vi "Initialize.vi"(8 "error in (no error)":errorcluster, 11 "Controller Actor.lvlib:Controller.lvclass":refnum<class "Controller.lvclass">) -> (0 "error out":errorcluster, 3 "Controller out":refnum<class "Controller.lvclass">)   [LabVIEW 2016, in "Controller Actor.lvlib" / "Controller.lvclass"]
uses:
  Controller.lvclass
  C:/Program Files (x86)/National Instruments/LabVIEW 2016/vi.lib/ActorFramework/Actor/Actor.lvclass
  <vilib>/ActorFramework/Actor/Actor.lvclass/Actor.ctl
  <vilib>/ActorFramework/Message Enqueuer/Message Enqueuer.lvclass/Message Enqueuer.ctl
  <vilib>/ActorFramework/Message Enqueuer/Init from Existing Queue.vi
  <vilib>/ActorFramework/Message Enqueuer/Enqueue.vi
  Messages/Measurements Scan Msg/Measurements Scan Msg.lvclass
  C:/Program Files (x86)/National Instruments/LabVIEW 2016/vi.lib/ActorFramework/Message/Message.lvclass
  <vilib>/ActorFramework/Message Priority Queue/Priority Enqueue.vi
  <vilib>/ActorFramework/Message Enqueuer/Message Enqueuer.lvclass
  <vilib>/ActorFramework/Actor/Actor.lvclass
  Messages/Scan Hardware Message/Scan Hardware Message.lvclass
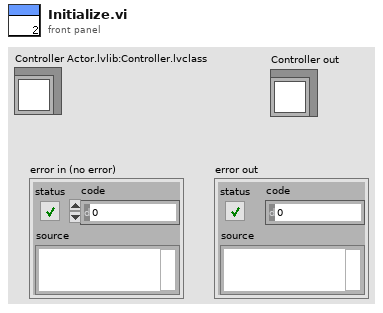
[diagram p1: front panel]
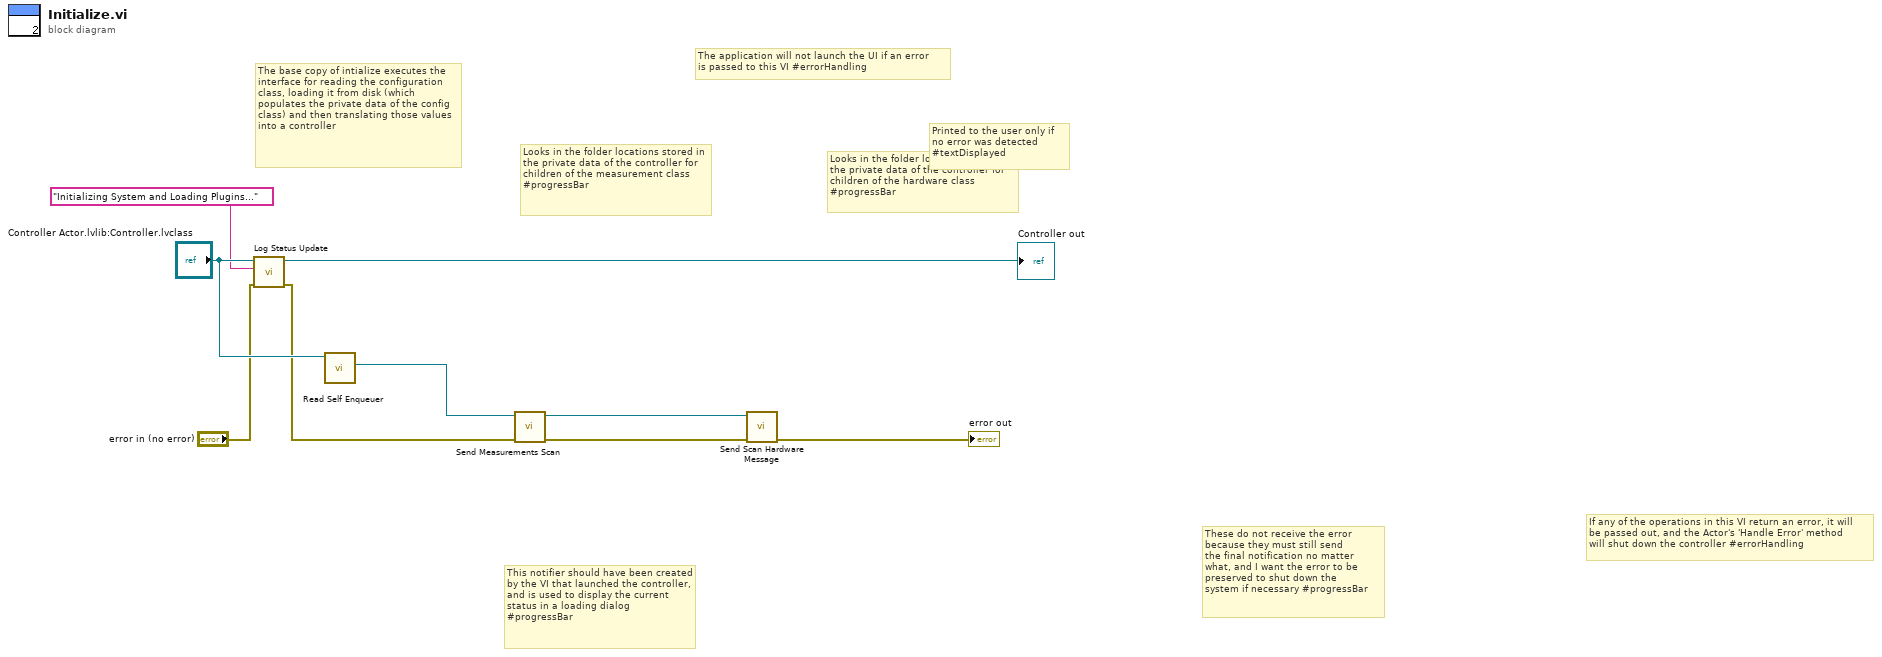
[diagram p0: block diagram]
diagram:
  # "The base copy of intialize executes the interface for reading the configuration class, loading it from disk (which populates the private data of the config class) and then translating those values into a controller"
  # "Printed to the user only if \nno error was detected\n#textDisplayed"
  # "This notifier should have been created by the VI that launched the controller, and is used to display the current status in a loading dialog #progressBar"
  # "Looks in the folder locations stored in the private data of the controller for children of the hardware class \n#progressBar"
  # "Looks in the folder locations stored in the private data of the controller for children of the measurement class #progressBar"
  # "These do not receive the error\nbecause they must still send \nthe final notification no matter \nwhat, and I want the error to be \npreserved to shut down the \nsystem if necessary #progressBar"
  # "The application will not launch the UI if an error\nis passed to this VI #errorHandling"
  # "If any of the operations in this VI return an error, it will\nbe passed out, and the Actor's 'Handle Error' method \nwill shut down the controller #errorHandling"
  n1 = call-dynamic "Log Status Update.vi"("error in (no error)"="error in (no error)", "String"="Initializing System and Loading Plugins...", "Controller in"="Controller Actor.lvlib:Controller.lvclass") -> ("error out"=w4:errorcluster, "Controller out"=→"Controller out":refnum<class "Controller.lvclass">)  [unwired: 7 in]
  n2 = call <vilib>:"Read Self Enqueuer.vi"("Actor"="Controller Actor.lvlib:Controller.lvclass") -> ("Self Enqueuer"=w9:refnum<class "Message Enqueuer.lvclass">)  [unwired: 10 in]
  n3 = call "Send Measurements Scan.vi"("error in (no error)"=w4, "Message Enqueuer"=w9) -> ("error out"=w2:errorcluster, "Message Enqueuer out"=w8:refnum<class "Message Enqueuer.lvclass">)  [unwired: 8 in]
  n4 = call "Send Scan Hardware Message.vi"("error in (no error)"=w2, "Message Enqueuer in"=w8) -> ("error out"=→"error out":errorcluster)  [unwired: 8 in, 1 out]
